vi "Show Configuration.vi"(8 "error in (no error)":errorcluster, 11 "Configuration in":refnum<class "Configuration.lvclass">) -> (0 "error out":errorcluster, 3 "Configuration out":refnum<class "Configuration.lvclass">)   [LabVIEW 2019, in "Configuration.lvclass"]
uses:
  Configuration.lvclass
  Configuration.lvclass/Configuration.ctl
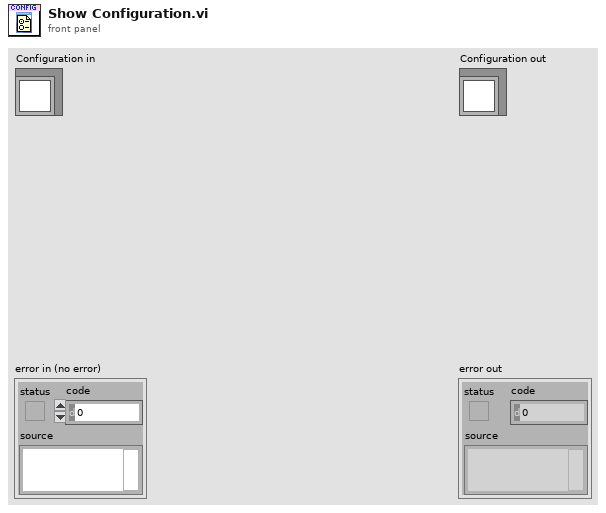
[diagram p1: front panel]
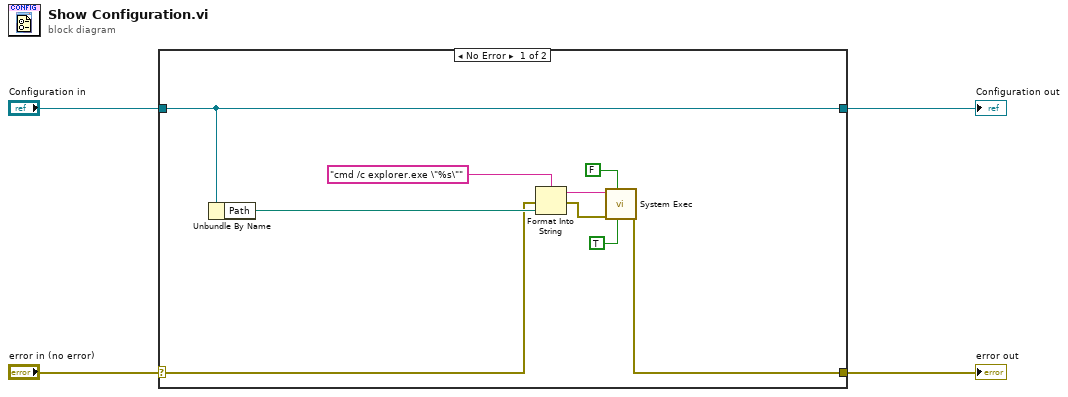
[diagram p0: block diagram]
diagram:
  n1 = case shown="No Error" "error in (no error)" {
    selector: "error in (no error)" -> [w8 w15]
    tunnel: [w7 w15] -> w1
    tunnel: [w13 w14] -> w4
    tunnel: "Configuration in" -> [w13 w14]
    frame No Error {
      n2 = Unbundle By Name(w13) -> ("Path"=w9:path)
      n3 = Format Into String(format string="cmd /c explorer.exe \"%s\"", error in=w8, w9) -> (resulting string=w11:string, error out=w10:errorcluster)  [unwired: 1 in]
      n4 = call <vilib>:"System Exec.vi"("run minimized? (F)"=TRUE, "wait until completion? (T)"=FALSE ("run minimized? (F)"), "error in (no error)"=w10, "command line"=w11) -> ("error out"=w7:errorcluster)  [unwired: 4 in, 3 out]
    }
    frame Error {
    }
  }
  "error out" <- w1
  "Configuration out" <- w4
